vi "ART-3029D-Set-DO.vi"(8 "error in (no error)":errorcluster, 10 "value":bool, 11 "DI":enum16{"DO0", "DO1", "DO2", "DO3", "DO4"}(ring)) -> (0 "error out":errorcluster)   [LabVIEW 2016, in "环境动力监测库.lvlib" / "浮标电源管理.lvlib"]
uses:
  <vilib>/Plasmionique/MB Master/MB_Master/MB_Master.lvclass
  <vilib>/Plasmionique/MB Master/MB Master.lvlib
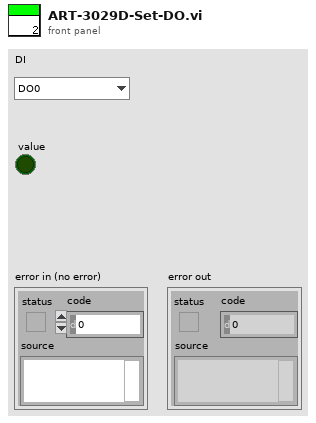
[diagram p1: front panel]
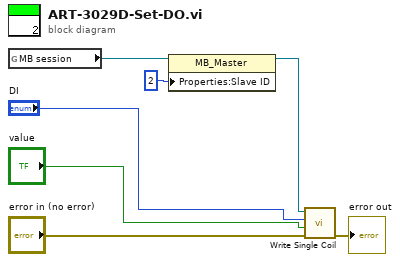
[diagram p0: block diagram]
diagram:
  n1 = global read "通讯全局变量.vi" "MB session"() -> (w4:refnum<class "MB_Master.lvclass">)
  n2 = property class="MB_Master"(reference=w4, "Properties:Slave ID"=u8 2 ("Slave ID")) -> (reference out=w3:refnum<class "MB_Master.lvclass">)  [unwired: 1 in, 1 out]
  n3 = call <vilib>:"Write Single Coil.vi"("error in (no error)"="error in (no error)", "value"="value", "address"="DI", "MB session in"=w3) -> ("error out"=→"error out":errorcluster)  [unwired: 6 in, 1 out]
